vi "GlobalCfg.vi"() -> ()   [LabVIEW 2014]
panel:
  in  "PPThomePos2":sgl format="%.2f"
  in  "PrgTypeID":i32 caption="产品识别代码："
  in  "CustomerNumber":i32 caption="产品识别代码："
  out "PProDataLog":bool
  in  "LogDays":dbl=100.0
  in  "PPTUNEnAn":sgl format="%.2f"
  in  "LOG_filePath":string="E:\\DATA\\"
  in  "Remote Port":u16=2080
  in  "Remote Host":string="10.2.20.80" caption="远程主机"
  in  "PArrayPT":sgl[][](array[numeric])=[[0.0, 0.0], [0.0, 0.0], [0.0, 0.0]] format="%.2f"
  in  "PPTHomeingSp":sgl format="%.2f"
  in  "PPTEnSwTr":i16
  in  "PPTEnSwSp":sgl format="%.2f"
  in  "PPTEnSwAng":sgl format="%.2f"
  in  "PPThomePos":sgl format="%.2f"
  in  "PPTStd":T1 {"PZBPTCCWAImT" format="%.2f"; "PZBPTCCWALoT" format="%.2f"; "PZBPTCCWAHiT" format="%.2f"; "PZBPTCCWVarT" format="%.2f"; "PZBPTCCWLoT" format="%.2f"; "PZBPTCCWHiT" format="%.2f"; "PZBPTCWALoT" format="%.2f"; "PZBPTCWAHiT" format="%.2f"; "PZBPTCWVarT" format="%.2f"; "PZBPTCWLoT" format="%.2f"; "PZBPTCWHiT" format="%.2f"; "PZAPTCCWAImT" format="%.2f"; "PZAPTCCWALoT" format="%.2f"; "PZAPTCCWAHiT" format="%.2f"; "PZAPTCCWVarT" format="%.2f"; "PZAPTCCWLoT" format="%.2f"; "PZAPTCCWHiT" format="%.2f"; "PZAPTCWALoT" format="%.2f"; "PZAPTCWAHiT" format="%.2f"; "PZAPTCWVarT" format="%.2f"; "PZAPTCWLoT" format="%.2f"; "PZAPTCWHiT" format="%.2f"}
  in  "PPTZone":T2 {"PZBPTendPOS" format="%.2f"; "PZBPTstPOS" format="%.2f"; "PZAPTendPOS" format="%.2f"; "PZAPTstPOS" format="%.2f"}
  in  "PPToffsetCCW":sgl format="%.2f"
  in  "PPToffsetCW":sgl format="%.2f"
  in  "PRPZone":T3 {"PZBRPendPOS" format="%.2f"; "PZBRPstPOS" format="%.2f"; "PZARPendPOS" format="%.2f"; "PZARPstPOS" format="%.2f"}
  in  "PRPStd":T4 {"PZBRPCCWAImF" format="%.2f"; "PZBRPCCWALoF" format="%.2f"; "PZBRPCCWAHiF" format="%.2f"; "PZBRPCCWVarF" format="%.2f"; "PZBRPCCWLoF" format="%.2f"; "PZBRPCCWHiF" format="%.2f"; "PZBRPCWALoF" format="%.2f"; "PZBRPCWAHiF" format="%.2f"; "PZBRPCWVarF" format="%.2f"; "PZBRPCWLoF" format="%.2f"; "PZBRPCWHiF" format="%.2f"; "PZARPCCWAImF" format="%.2f"; "PZARPCCWALoF" format="%.2f"; "PZARPCCWAHiF" format="%.2f"; "PZARPCCWVarF" format="%.2f"; "PZARPCCWLoF" format="%.2f"; "PZARPCCWHiF" format="%.2f"; "PZARPCWALoF" format="%.2f"; "PZARPCWAHiF" format="%.2f"; "PZARPCWVarF" format="%.2f"; "PZARPCWLoF" format="%.2f"; "PZARPCWHiF" format="%.2f"}
  in  "PRPoffsetR":sgl format="%.2f"
  in  "PRPoffsetL":sgl format="%.2f"
  in  "PmaxNOLdist":sgl format="%.2f"
  in  "PAbCenterPos":sgl format="%.2f"
  in  "PArrayRP":sgl[][](array[numeric])=[[0.0, 0.0, 0.0, 0.0, 0.0, 0.0, 0.0, 0.0], [0.0, 0.0, 0.0, 0.0, 0.0, 0.0, 0.0, 0.0], [0.0, 0.0, 0.0, 0.0, 0.0, 0.0, 0.0, 0.0]] format="%.2f"
  in  "PFailAbort":i32
  in  "PRPEcycle":i32
  in  "PGearRatio":sgl format="%.2f"
  in  "PRack_Lock2Lock":sgl format="%.2f"
  out "currentTID":i32
  in  "TestSpec":string="VWCII38HE-1612links" caption="Test specification:"
  in  "TypeNumber":string="32035552PEP" caption="Type number:"
  out "typelist":string[](array[string])
  out "TotalType":i32
  out "currentType":string
  # "系统自用参数,用修改配置文件方法修改"
  # "Rotate\nto right"
  # "Rotate\nto left"
  # "angle\n\nSpeed\n\nOverload"
  # "Right\nEnd"
  # "Left\nstart"
  # "Left\nend"
  # "Right\nstart"
  # "Right\nEnd"
  # "Home"
  # "Home"
  # "Centering"
  # "position\n\nSpeed\n\nOverload"
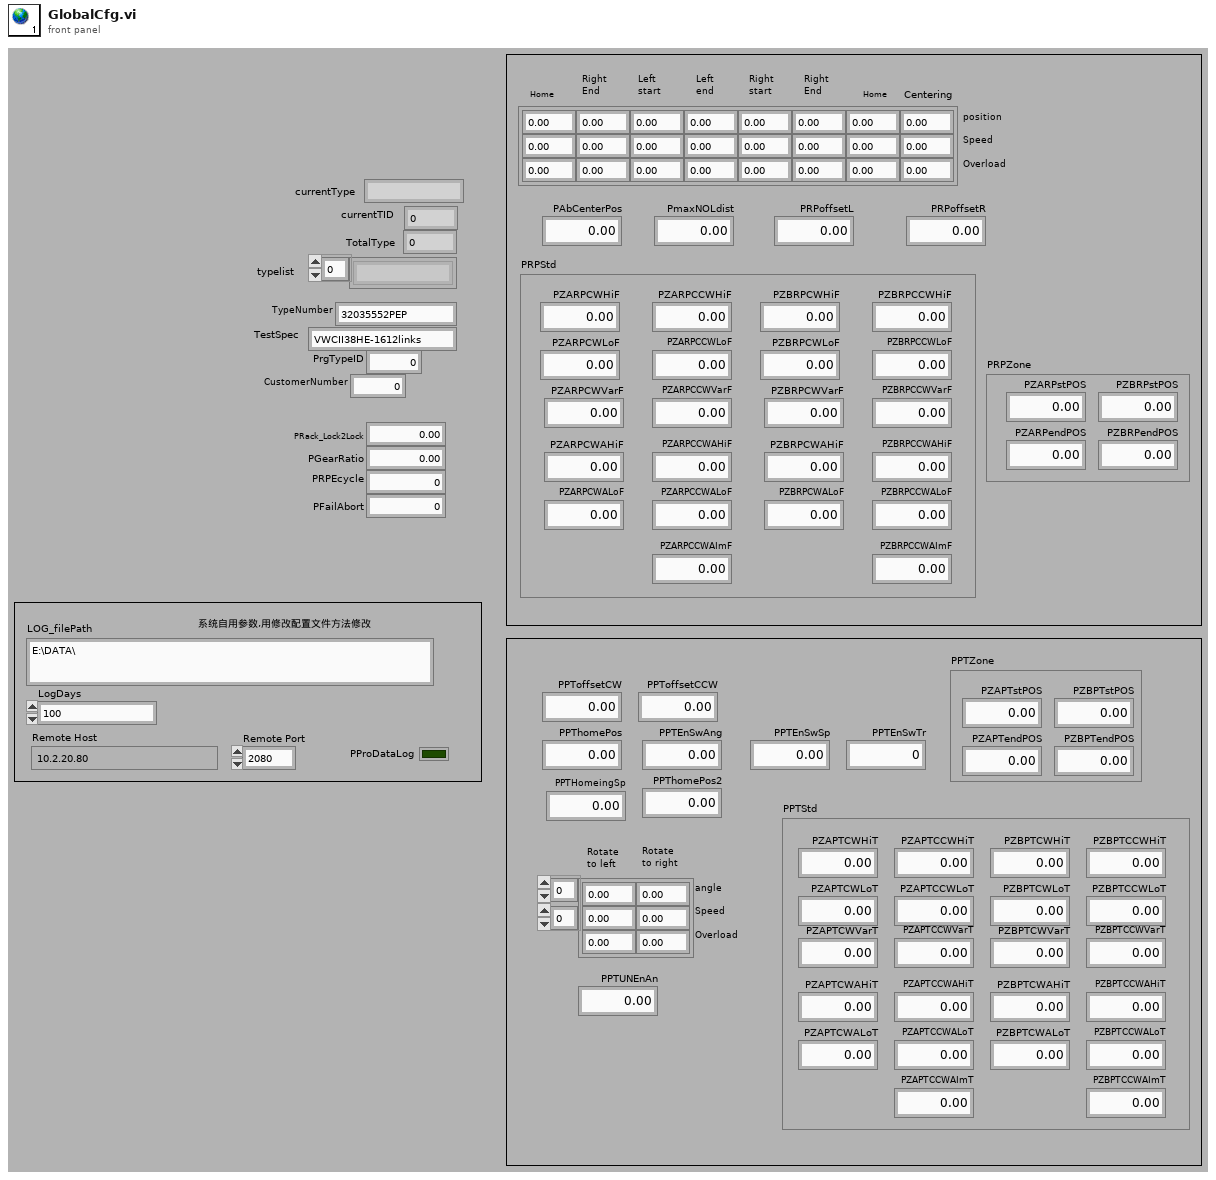
[diagram p1: front panel]
types:
  T1 = cluster{"PZAPTCWHiT":sgl, "PZAPTCWLoT":sgl, "PZAPTCWVarT":sgl, "PZAPTCWAHiT":sgl, "PZAPTCWALoT":sgl, "PZAPTCCWHiT":sgl, "PZAPTCCWLoT":sgl, "PZAPTCCWVarT":sgl, "PZAPTCCWAHiT":sgl, "PZAPTCCWALoT":sgl, "PZAPTCCWAImT":sgl, "PZBPTCWHiT":sgl, "PZBPTCWLoT":sgl, "PZBPTCWVarT":sgl, "PZBPTCWAHiT":sgl, "PZBPTCWALoT":sgl, "PZBPTCCWHiT":sgl, "PZBPTCCWLoT":sgl, "PZBPTCCWVarT":sgl, "PZBPTCCWAHiT":sgl, "PZBPTCCWALoT":sgl, "PZBPTCCWAImT":sgl}
  T2 = cluster{"PZAPTstPOS":sgl, "PZAPTendPOS":sgl, "PZBPTstPOS":sgl, "PZBPTendPOS":sgl}
  T3 = cluster{"PZARPstPOS":sgl, "PZARPendPOS":sgl, "PZBRPstPOS":sgl, "PZBRPendPOS":sgl}
  T4 = cluster{"PZARPCWHiF":sgl, "PZARPCWLoF":sgl, "PZARPCWVarF":sgl, "PZARPCWAHiF":sgl, "PZARPCWALoF":sgl, "PZARPCCWHiF":sgl, "PZARPCCWLoF":sgl, "PZARPCCWVarF":sgl, "PZARPCCWAHiF":sgl, "PZARPCCWALoF":sgl, "PZARPCCWAImF":sgl, "PZBRPCWHiF":sgl, "PZBRPCWLoF":sgl, "PZBRPCWVarF":sgl, "PZBRPCWAHiF":sgl, "PZBRPCWALoF":sgl, "PZBRPCCWHiF":sgl, "PZBRPCCWLoF":sgl, "PZBRPCCWVarF":sgl, "PZBRPCCWAHiF":sgl, "PZBRPCCWALoF":sgl, "PZBRPCCWAImF":sgl}
diagram:
